vi "5492_WPI_RobotDriveMotors.vi"(8 "error in (no error)":errorcluster, 9 "RightSpeed":dbl, 10 "LeftSpeed":dbl, 11 "RobotDriveDevRef":T1={"DevStatus"={"status"=FALSE, "code"=0, "source"=""}, "Motors[]"=[], "Square Inputs"=FALSE, "Max Output"=1.0}) -> (0 "error out":errorcluster, 2 "Motor Values":dbl[](array[numeric]), 3 "RobotDriveDevRef":T1={"DevStatus"={"status"=FALSE, "code"=0, "source"=""}, "Motors[]"=[], "Square Inputs"=FALSE, "Max Output"=1.0})   [LabVIEW 2016]
doc: "Determines the motor configuration and sends the speed values to the appropriate motors.\n\nThis software is licensed. Open the labview\\readme\\WPI Robotics Library Open Source License.txt file for more information."
uses:
  <vilib>/Rock Robotics/WPI/RobotDrive/WPI_RobotDriveDevRef.ctl
  <vilib>/Rock Robotics/WPI/MotorControl/WPI_MotorControlDeviceRef.ctl
  <vilib>/Rock Robotics/WPI/MotorControl/WPI_MotorControlType.ctl
  <vilib>/Rock Robotics/SystemInterfaces/DIO/FPGA_DIOPWMChannel.ctl
  <vilib>/Rock Robotics/WPI/PWM/WPI_PWMDeadband.ctl
  5492_WPI_RobotDriveMotorSelectorEnum.ctl
  <vilib>/Rock Robotics/WPI/RobotDrive/WPI_RobotDriveSafetyCheck.vi
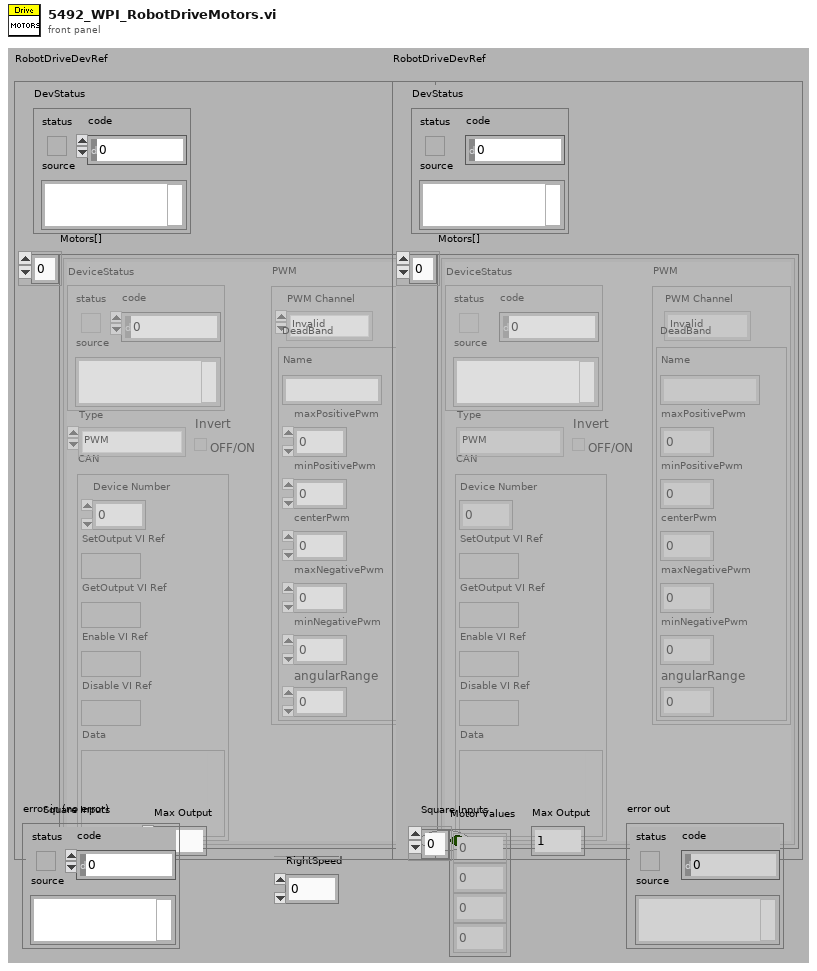
[diagram p1: front panel]
types:
  T1 = typedef "WPI_RobotDriveDevRef.ctl" = cluster{"DevStatus":errorcluster, "Motors[]":T2[], "Square Inputs":bool, "Max Output":dbl}
  T2 = typedef "WPI_MotorControlDeviceRef.ctl" = cluster{"DeviceStatus":errorcluster, "Type":T3, "PWM":cluster{"PWM Channel":T4, "DeadBand":T5}, "CAN":cluster{"Device Number":u8, "SetOutput VI Ref":variant, "GetOutput VI Ref":variant, "Enable VI Ref":variant, "Disable VI Ref":variant, "Data":variant}, "Invert":bool}
  T3 = typedef "WPI_MotorControlType.ctl" = enum16{"PWM", "CAN"}
  T4 = typedef "FPGA_DIOPWMChannel.ctl" = enum8{"PWM 0", "PWM 1", "PWM 2", "PWM 3", "PWM 4", "PWM 5", "PWM 6", "PWM 7", "PWM 8", "PWM 9", "PWM MXP 0", "PWM MXP 1", "PWM MXP 2", "PWM MXP 3", "PWM MXP 4", "PWM MXP 5", "PWM MXP 6", "PWM MXP 7", "PWM MXP 8", "PWM MXP 9", "Invalid"}
  T5 = typedef "WPI_PWMDeadband.ctl" = cluster{"Name":string, "maxPositivePwm":i32, "minPositivePwm":i32, "centerPwm":i32, "maxNegativePwm":i32, "minNegativePwm":i32, "angularRange":u16}
  T6 = typedef "5492_WPI_RobotDriveMotorSelectorEnum.ctl" = enum16{"Front left motor", "Front right motor", "Back left motor", "Back right motor"}
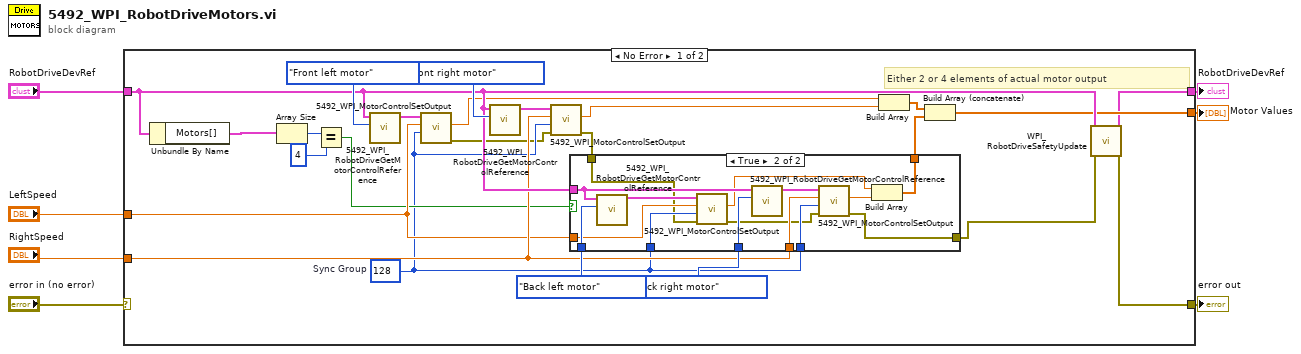
[diagram p0: block diagram]
diagram:
  n1 = case shown="No Error" "error in (no error)" {
    selector: "error in (no error)" -> [_ w49]
    tunnel: "RobotDriveDevRef" -> [w23 w48]
    tunnel: [w8 w48] -> w6
    tunnel: "LeftSpeed" -> [w21 _]
    tunnel: "RightSpeed" -> [w22 _]
    tunnel: [w9 w49] -> w2
    tunnel: [w11 _] -> w1
    frame No Error {
      w19 = u8 128  # Sync Group
      # "Either 2 or 4 elements of actual motor output"
      n2 = Unbundle By Name(w23) -> ("Motors[]"=w18:T2[])
      n3 = Array Size(array=w18) -> (size(s)=w31:i32)
      n4 = Equal?(x=w31, y=4) -> (x = y?=w20:bool)
      n5 = call "5492_WPI_RobotDriveGetMotorControlReference.vi"("MotorIndex"=5492_WPI_RobotDriveMotorSelectorEnum."Front left motor", "RobotDriveDevRef"=w23) -> ("MotorControlDeviceRef"=w28:T2)  [unwired: 9 out]
      n6 = call "5492_WPI_MotorControlSetOutput.vi"("options"=w19, "Output"=w21, "MotorControlDevRef"=w28) -> ("error out"=w17:errorcluster, "Motor Output"=w15:dbl)  [unwired: 2 in, 5 out]
      n7 = call "5492_WPI_RobotDriveGetMotorControlReference.vi"("MotorIndex"=5492_WPI_RobotDriveMotorSelectorEnum."Front right motor", "RobotDriveDevRef"=w23) -> ("MotorControlDeviceRef"=w29:T2)  [unwired: 9 out]
      n8 = call "5492_WPI_MotorControlSetOutput.vi"("error in (no error)"=w17, "options"=w19, "Output"=w22, "MotorControlDevRef"=w29) -> ("error out"=w16:errorcluster, "Motor Output"=w14:dbl)  [unwired: 1 in, 5 out]
      n9 = case shown="True" w20 {
        tunnel: 5492_WPI_RobotDriveMotorSelectorEnum."Back left motor" ("MotorIndex") -> [_ w47]
        tunnel: 5492_WPI_RobotDriveMotorSelectorEnum."Back right motor" ("MotorIndex") -> [_ w46]
        tunnel: w23 -> [_ w45]
        tunnel: w19 -> [_ w44]
        tunnel: w22 -> [_ w43]
        tunnel: w21 -> [_ w42]
        tunnel: [w32 w38] -> w10
        tunnel: w19 -> [_ w39]
        tunnel: w16 -> [w32 w36]
        tunnel: [_ w33] -> w13
        frame False {
        }
        frame True {
          n10 = call "5492_WPI_RobotDriveGetMotorControlReference.vi"("MotorIndex"=w47, "RobotDriveDevRef"=w45) -> ("MotorControlDeviceRef"=w40:T2)  [unwired: 9 out]
          n11 = call "5492_WPI_MotorControlSetOutput.vi"("error in (no error)"=w36, "options"=w39, "Output"=w42, "MotorControlDevRef"=w40) -> ("error out"=w37:errorcluster, "Motor Output"=w34:dbl)  [unwired: 1 in, 5 out]
          n12 = call "5492_WPI_RobotDriveGetMotorControlReference.vi"("MotorIndex"=w46, "RobotDriveDevRef"=w45) -> ("MotorControlDeviceRef"=w41:T2)  [unwired: 9 out]
          n13 = call "5492_WPI_MotorControlSetOutput.vi"("error in (no error)"=w37, "options"=w44, "Output"=w43, "MotorControlDevRef"=w41) -> ("error out"=w38:errorcluster, "Motor Output"=w35:dbl)  [unwired: 1 in, 5 out]
          n14 = Build Array(w34, w35) -> (w33:dbl[])
        }
      }
      n15 = Build Array(w15, w14) -> (w12:dbl[])
      n16 = Build Array (concatenate)(w12, w13) -> (w11:dbl[])
      n17 = call <vilib>:"WPI_RobotDriveSafetyUpdate.vi"("error in (no error)"=w10, "RobotDriveDevRef"=w23) -> ("error out"=w9:errorcluster, "RobotDriveDevRef"=w8:T1)  [unwired: 8 out]
    }
    frame Error {
    }
  }
  "RobotDriveDevRef" <- w6
  "error out" <- w2
  "Motor Values" <- w1
